vi "FT10_Unitherm Set Load.vi"(8 "error in (no error)":errorcluster, 10 "Load Impedance":i32 max=6400 step=1, 11 "VISA Refnum in":refnum<visa-resource-name>) -> (0 "error out":errorcluster, 3 "VISA Refnum out":refnum<visa-resource-name>)   [LabVIEW 2015]
doc: "Adjusts impedance on Unitherm to value received at Load Impedance control."
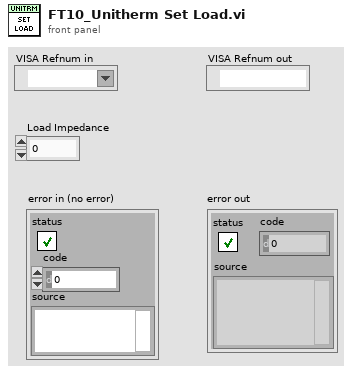
[diagram p1: front panel]
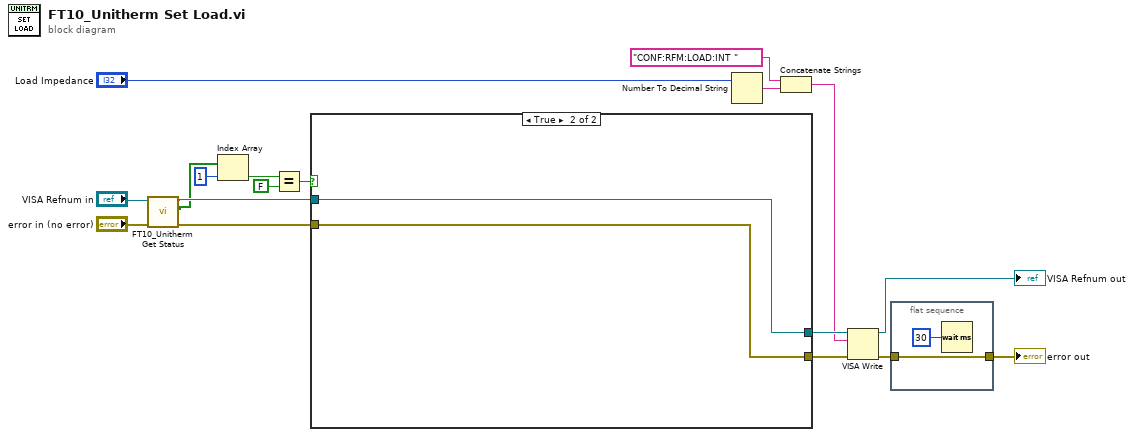
[diagram p0: block diagram]
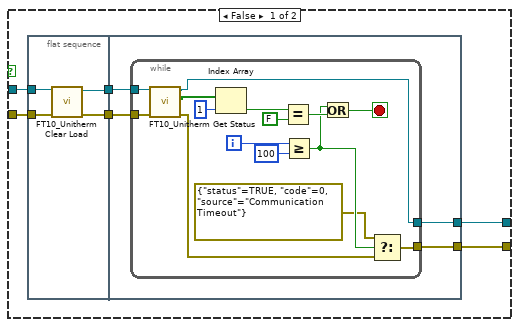
[diagram p2: hidden frame]
diagram:
  n1 = call "FT10_Unitherm Get Status.vi"("error in (no error)"="error in (no error)", "VISA Refnum in"="VISA Refnum in") -> ("error out"=w14:errorcluster, "Status"=w15:bool[], "VISA Refnum out"=w16:refnum<visa-resource-name>)  [unwired: 7 in]
  n2 = Index Array(array=w15, index=1) -> (element=w10:bool)
  n3 = Equal?(x=w10, y=FALSE) -> (x = y?=w9:bool)
  n4 = case shown="True" w9 {
    tunnel: w16 -> [w24 w49]
    tunnel: [w21 w49] -> w5
    tunnel: w14 -> [w23 w48]
    tunnel: [w22 w48] -> w6
    frame False {
      n5 = flat-sequence {
        tunnel: w24 -> [w28]
        tunnel: w23 -> [w25]
        tunnel: [w26] -> w20
        tunnel: [w27] -> w19
        tunnel: w20 -> [w32]
        tunnel: w19 -> [w30]
        tunnel: [w31] -> w22
        tunnel: [w29] -> w21
        frame #0 {
          n6 = call "FT10_Unitherm Clear Load.vi"("error in (no error)"=w25, "VISA Refnum in"=w28) -> ("error out"=w26:errorcluster, "VISA Refnum out"=w27:refnum<visa-resource-name>)  [unwired: 8 in]
        }
        frame #1 {
          n7 = while {
            tunnel: w32 -> [w34]
            tunnel: [w41] -> w31
            tunnel: w30 -> [w33]
            tunnel: [w37] -> w29
            i -> [w45]
            stop <- w47 stop-if-true
            n8 = call "FT10_Unitherm Get Status.vi"("error in (no error)"=w34, "VISA Refnum in"=w33) -> ("error out"=w35:errorcluster, "Status"=w36:bool[], "VISA Refnum out"=w37:refnum<visa-resource-name>)  [unwired: 7 in]
            n9 = Index Array(array=w36, index=1) -> (element=w39:bool)
            n10 = Equal?(x=w39, y=FALSE) -> (x = y?=w46:bool)
            n11 = Greater Or Equal?(x=w45, y=100 ("x")) -> (x >= y?=w43:bool)
            n12 = Or(x=w43, y=w46) -> (x .or. y?=w47:bool)
            n13 = Select(t=errorcluster {"status"=TRUE, "code"=0, "source"="Communication Timeout"} ("error out"), s=w43, f=w35) -> (s? t:f=w41:errorcluster)
          }
        }
      }
    }
    frame True {
    }
  }
  n14 = Number To Decimal String(number="Load Impedance") -> (decimal integer string=w3:string)  [unwired: 1 in]
  n15 = Concatenate Strings("CONF:RFM:LOAD:INT " ("string"), w3) -> (w4:string)
  n16 = VISA Write(VISA resource name=w5, write buffer=w4, error in (no error)=w6) -> (VISA resource name out=→"VISA Refnum out":refnum<visa-resource-name>, error out=w12:errorcluster)  [unwired: 1 out]
  n17 = flat-sequence {
    tunnel: w12 -> [w50]
    tunnel: [w50] -> w13
    frame #0 {
      n18 = Wait (ms)(milliseconds to wait=u32 30) -> ()  [unwired: 1 out]
    }
  }
  "error out" <- w13
